vi "niRFUtil WFM Correlate (complex wfm).vi"(1 "Reference Waveform* In":T1 {"y" format="%.2f"; "dx" format="%^.2e"; "x0" format="%^.2e"}, 2 "Waveform In":T1 {"y" format="%.2f"; "dx" format="%^.2e"; "x0" format="%^.2e"}) -> (0 "Waveform Out":T1 {"y" format="%.2f"; "dx" format="%^.2e"; "x0" format="%^.2e"})   [LabVIEW 2015, in "niRFUtil.lvlib"]
doc: "(c) Copyright 2006, National Instruments, Inc. This VI may not be duplicated, sold, or distributed without written consent from National Instruments."
uses:
  niRFUtil.lvlib
  Includes/niRFUtil INC Complex Waveform.ctl
  Includes/niRFUtil INC Complex Array.ctl
  <vilib>/Analysis/2dsp.llb/1D Cross Correlation (CDB).vi
  <vilib>/Analysis/NI_AALPro.lvlib
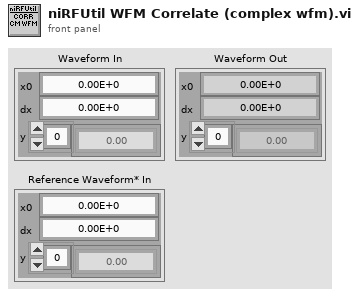
[diagram p1: front panel]
types:
  T1 = typedef "niRFUtil.lvlib/niRFUtil INC Complex Waveform.ctl" = cluster{"x0":dbl, "dx":dbl, "y":T2}
  T2 = typedef "niRFUtil.lvlib/niRFUtil INC Complex Array.ctl" = csg[]
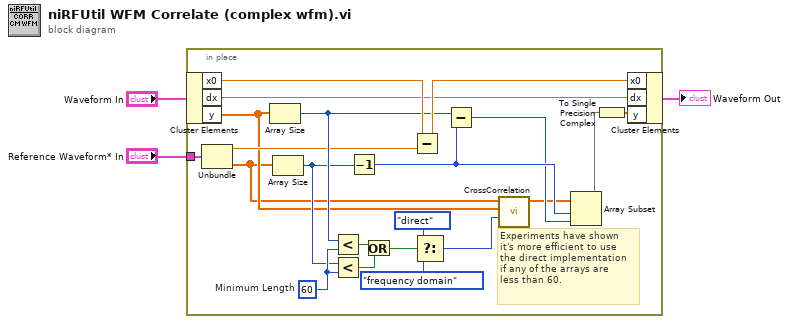
[diagram p0: block diagram]
diagram:
  n1 = in-place {
    in-place-border: "Reference Waveform* In" -> [w10]
    w24 = 60  # Minimum Length
    # "Experiments have shown\nit's more efficient to use\nthe direct implementation\nif any of the arrays are\nless than 60."
    n2 = in-place-cluster #1("Waveform In") -> ("x0"=w18:dbl, "dx"=w15:dbl, "y"=w6:T2)
    n3 = Unbundle(w10) -> ("x0"=w9:dbl, "y"=w5:T2)  [unwired: 1 out]
    n4 = Array Size(array=w6) -> (size(s)=w12:i32)
    n5 = Array Size(array=w5) -> (size(s)=w11:i32)
    n6 = Less?(x=w12, y=w24) -> (x < y?=w23:bool)
    n7 = Less?(x=w11, y=w24) -> (x < y?=w22:bool)
    n8 = Decrement(x=w11) -> (x-1=w14:i32)
    n9 = Or(x=w23, y=w22) -> (x .or. y?=w21:bool)
    n10 = Subtract(x=w18, y=w9) -> (x-y=w17:dbl)
    n11 = Select(t=enum32{"direct", "frequency domain"}."direct" ("algorithm"), s=w21, f=enum32{"direct", "frequency domain"}."frequency domain" ("algorithm")) -> (s? t:f=w4:enum32{"direct", "frequency domain"})
    n12 = Subtract(x=w12, y=w14) -> (x-y=w13:i32)
    n13 = call-poly <vilib>:"CrossCorrelation.vi"("algorithm"=w4, "Y"=w6, "X"=w5) -> ("Rxy"=w7:cdb[])  [unwired: 7 in, 1 out]
    n14 = Array Subset(array=w7, index=w14, length=w13) -> (w16:cdb[])
    n15 = To Single Precision Complex(1:w16) -> (0:w8:csg[])
    n16 = in-place-cluster #1("x0"=w17, "dx"=w15, "y"=w8) -> (→"Waveform Out":T1)
  }
